vi "CRYItemCheckSort.vi"(9 "Check_s":bool[](array[boolean]), 11 "In Items":string[](array[string])) -> (0 "Out Check":bool[](array[boolean]), 1 "Out Items":string[](array[string]), 2 "Unchk Items":string[](array[string]), 3 "Chked Items":string[](array[string]))   [LabVIEW 2013]
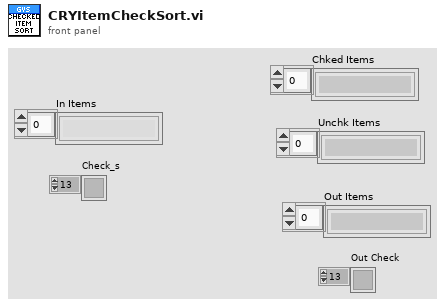
[diagram p1: front panel]
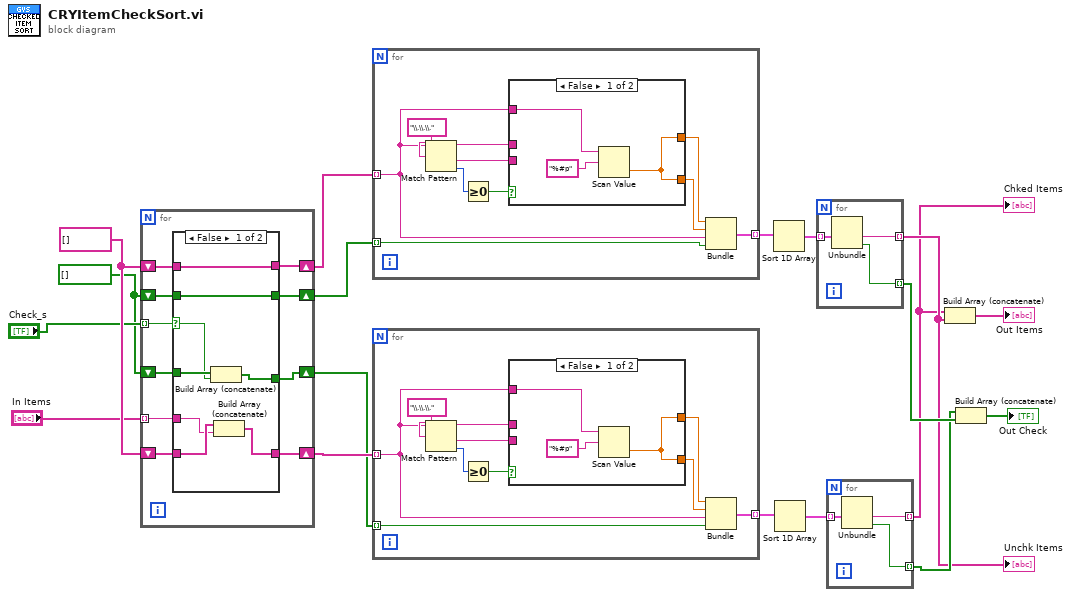
[diagram p0: block diagram]
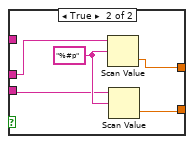
[diagram p2: hidden frame]
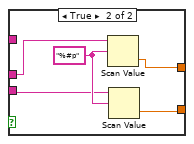
[diagram p3: hidden frame]
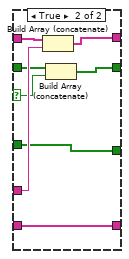
[diagram p4: hidden frame]
diagram:
  w7 = bool[] [] ("Array")
  w18 = string[] [] ("Array")
  n1 = for {
    tunnel: "Check_s" -> [w19] mode=indexing
    tunnel: "In Items" -> [w26] mode=indexing
    shift-right: [w28] -> w17
    shift-left: w18 -> [w27]
    shift-right: [w25] -> w12
    shift-left: w18 -> [w24]
    shift-right: [w23] -> w8
    shift-left: w7 -> [w22]
    shift-right: [w21] -> w6
    shift-left: w7 -> [w20]
    n2 = case shown="False" w19 {
      selector: w19 -> [w31 w38]
      tunnel: [w36 w42] -> w28
      tunnel: w27 -> [w36 w43]
      tunnel: w26 -> [w34 w44]
      tunnel: [w33 w41] -> w25
      tunnel: w24 -> [w35 w41]
      tunnel: [w29 w39] -> w23
      tunnel: w22 -> [w29 w40]
      tunnel: [w30 w37] -> w21
      tunnel: w20 -> [w32 w37]
      frame False {
        n3 = Build Array (concatenate)(w32, w31) -> (w30:bool[])
        n4 = Build Array (concatenate)(w35, w34) -> (w33:string[])
      }
      frame True {
        n5 = Build Array (concatenate)(w43, w44) -> (w42:string[])
        n6 = Build Array (concatenate)(w40, w38) -> (w39:bool[])
      }
    }
  }
  n7 = for {
    tunnel: w17 -> [w51] mode=indexing
    tunnel: [w50] -> w15 mode=indexing
    tunnel: w8 -> [w45] mode=indexing
    n8 = Match Pattern(string=w51, regular expression="\\.\\.\\.") -> (before substring=w49:string, after substring=w48:string, offset past match=w54:i32)  [unwired: 2 out]
    n9 = Greater Or Equal To 0?(x=w54) -> (x >= 0?=w53:bool)
    n10 = case shown="False" w53 {
      tunnel: w51 -> [w57 _]
      tunnel: [w55 w59] -> w47
      tunnel: w49 -> [_ w61]
      tunnel: w48 -> [_ w60]
      tunnel: [w55 w58] -> w46
      frame False {
        n11 = Scan Value(string=w57, format string="%#p") -> (value=w55:dbl)  [unwired: 1 in, 1 out]
      }
      frame True {
        w62 = "%#p" ("format string")
        n12 = Scan Value(string=w61, format string=w62) -> (value=w59:dbl)  [unwired: 1 in, 1 out]
        n13 = Scan Value(string=w60, format string=w62) -> (value=w58:dbl)  [unwired: 1 in, 1 out]
      }
    }
    n14 = Bundle(w47, w46, w51, w45) -> (w50:cluster{dbl, dbl, string, bool})  [unwired: 1 out]
  }
  n15 = for {
    tunnel: w12 -> [w69] mode=indexing
    tunnel: w6 -> [w68] mode=indexing
    tunnel: [w67] -> w13 mode=indexing
    n16 = Match Pattern(string=w69, regular expression="\\.\\.\\.") -> (before substring=w66:string, after substring=w65:string, offset past match=w72:i32)  [unwired: 2 out]
    n17 = Greater Or Equal To 0?(x=w72) -> (x >= 0?=w71:bool)
    n18 = case shown="False" w71 {
      tunnel: w69 -> [w75 _]
      tunnel: [w73 w77] -> w64
      tunnel: w66 -> [_ w79]
      tunnel: w65 -> [_ w78]
      tunnel: [w73 w76] -> w63
      frame False {
        n19 = Scan Value(string=w75, format string="%#p") -> (value=w73:dbl)  [unwired: 1 in, 1 out]
      }
      frame True {
        w80 = "%#p" ("format string")
        n20 = Scan Value(string=w79, format string=w80) -> (value=w77:dbl)  [unwired: 1 in, 1 out]
        n21 = Scan Value(string=w78, format string=w80) -> (value=w76:dbl)  [unwired: 1 in, 1 out]
      }
    }
    n22 = Bundle(w64, w63, w69, w68) -> (w67:cluster{dbl, dbl, string, bool})  [unwired: 1 out]
  }
  n23 = Sort 1D Array(array=w15) -> (sorted array=w16:cluster{dbl, dbl, string, bool}[])
  n24 = Sort 1D Array(array=w13) -> (sorted array=w14:cluster{dbl, dbl, string, bool}[])
  n25 = for {
    tunnel: w16 -> [w83] mode=indexing
    tunnel: [w82] -> w2 mode=indexing
    tunnel: [w81] -> w4 mode=indexing
    n26 = Unbundle(w83) -> (w82:string, w81:bool)  [unwired: 2 out]
  }
  "Unchk Items" <- w2
  n27 = for {
    tunnel: w14 -> [w86] mode=indexing
    tunnel: [w85] -> w1 mode=indexing
    tunnel: [w84] -> w3 mode=indexing
    n28 = Unbundle(w86) -> (w85:string, w84:bool)  [unwired: 2 out]
  }
  "Chked Items" <- w1
  n29 = Build Array (concatenate)(w1, w2) -> (→"Out Items":string[])
  n30 = Build Array (concatenate)(w3, w4) -> (→"Out Check":bool[])
